vi "Write State.vi"(8 "error in (no error)":errorcluster, 10 "State":string, 11 "SPARC4_GEI in":refnum<class "S4GEI.lvclass">) -> (0 "error out":errorcluster, 3 "SPARC4_GEI out":refnum<class "S4GEI.lvclass">)   [LabVIEW 2018, in "S4GEI.lvclass"]
uses:
  S4GEI.lvclass
  S4GEI.lvclass/S4GEI.ctl
  State Machine/State Machine.lvclass
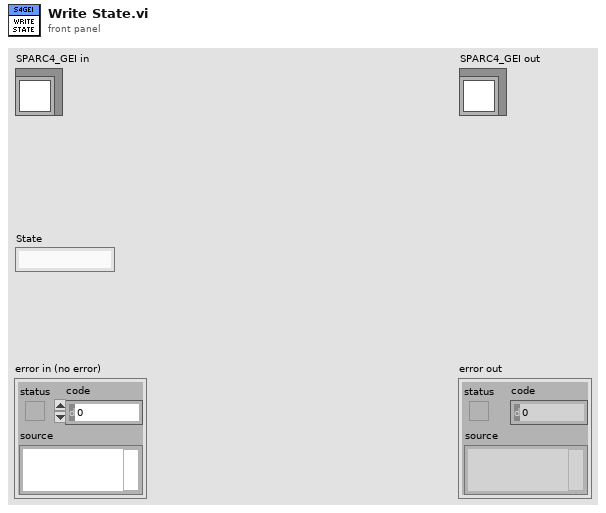
[diagram p1: front panel]
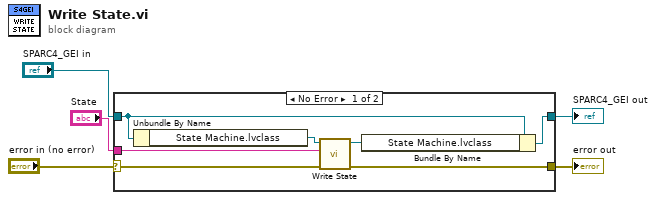
[diagram p0: block diagram]
diagram:
  n1 = case shown="No Error" "error in (no error)" {
    selector: "error in (no error)" -> [w10 w14]
    tunnel: [w9 w14] -> w4
    tunnel: [w11 w13] -> w2
    tunnel: "SPARC4_GEI in" -> [w12 w13]
    tunnel: "State" -> [w6 _]
    frame No Error {
      n2 = Unbundle By Name(w12) -> ("State Machine.lvclass"=w7:refnum<class "State Machine.lvclass">)
      n3 = call-dynamic "Write State.vi"("error in (no error)"=w10, "State"=w6, "State Machine in"=w7) -> ("error out"=w9:errorcluster, "State Machine out"=w8:refnum<class "State Machine.lvclass">)  [unwired: 7 in]
      n4 = Bundle By Name(cluster=w12, "State Machine.lvclass"=w8) -> (w11:refnum<class "S4GEI.lvclass">)
    }
    frame Error {
    }
  }
  "error out" <- w4
  "SPARC4_GEI out" <- w2
